vi "SRV_Display.vi"(0 "Variable Name":string="WORK1", 2 "SuperPro":T1) -> (4 "SuperPro":T1)   [LabVIEW 2009]
doc: "End the closest for loop"
uses:
  <userlib>/SuperPro/OpCodes/_SubVIs/SuperProControl.ctl
panel:
  # "This LabVIEW item is deprecated.\n\nIt is believed to be unused and will be removed in a future version of SRV."
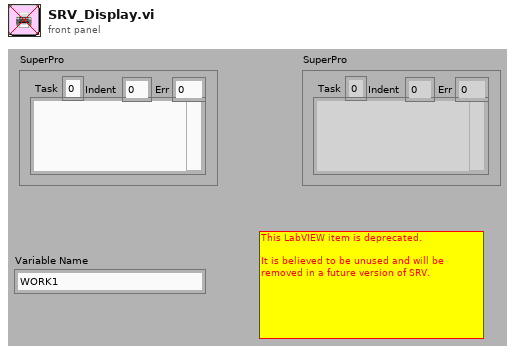
[diagram p1: front panel]
types:
  T1 = typedef "SuperProControl.ctl" = cluster{"Task":i32, "Indent":i32, "Err":i32, "ASM":string}
  T2 = enum16{"boolean", "u8", "i8", "u16", "i16", "u32", "i32", "u64", "i64", "SGL", "DBL", "EXT", "CPX"}
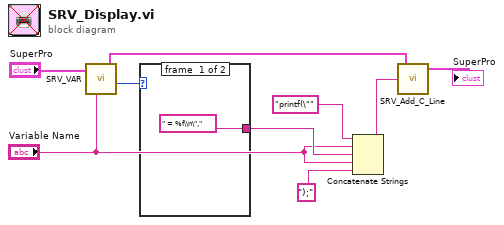
[diagram p0: block diagram]
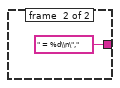
[diagram p2: hidden frame]
diagram:
  n1 = call "SRV_VAR.vi"("SuperPro in"="SuperPro", "Name"="Variable Name") -> ("SuperPro out"=w2:T1, "type out"=w5:T2)  [unwired: 1 in, 2 out]
  n2 = case shown="Default" w5 {
    tunnel: [" = %f\\n\"," ("format string") " = %d\\n\"," ("format string")] -> w4
    frame #0 {
    }
    frame #1 {
    }
  }
  n3 = Concatenate Strings("printf(\"" ("format string"), "Variable Name", w4, "Variable Name", ");" ("format string")) -> (w6:string)
  n4 = call "SRV_Add_C_Line.vi"("C String"=w6, "SuperPro in"=w2) -> ("SuperPro out"=→"SuperPro":T1)  [unwired: 3 in]
